vi "GetType.vi"(8 "error in (no error)":errorcluster, 11 "Stop Scan Msg":refnum<class "Stop Scan Msg.lvclass">) -> (0 "error out":errorcluster, 2 "Data Sample":variant, 3 "Stop Scan Msg":refnum<class "Stop Scan Msg.lvclass">)   [LabVIEW 2015, in "CS++MCS.lvlib" / "Stop Scan Msg.lvclass"]
uses:
  Stop Scan Msg.lvclass
  Stop Scan Msg.lvclass/Stop Scan Msg.ctl
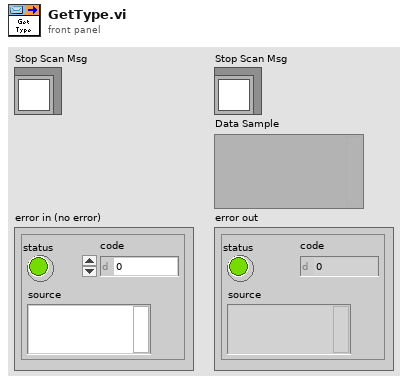
[diagram p1: front panel]
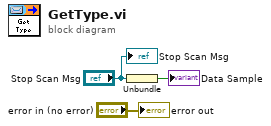
[diagram p0: block diagram]
diagram:
  n1 = Unbundle("Stop Scan Msg") -> (→"Data Sample":bool)
  "error out" <- "error in (no error)"
  "Stop Scan Msg" <- "Stop Scan Msg"
